vi "04 WriteOff.vi"(8 "error in (no error)":errorcluster caption="错误输入（无错误）", 11 "SerialClass 输入":refnum<class "SerialClass.lvclass">) -> (0 "error out":errorcluster caption="错误输出", 3 "SerialClass 输出":refnum<class "SerialClass.lvclass">)   [LabVIEW 2019, in "SerialClass.lvclass"]
uses:
  SerialClass.lvclass
  SerialClass.lvclass/SerialClass.ctl
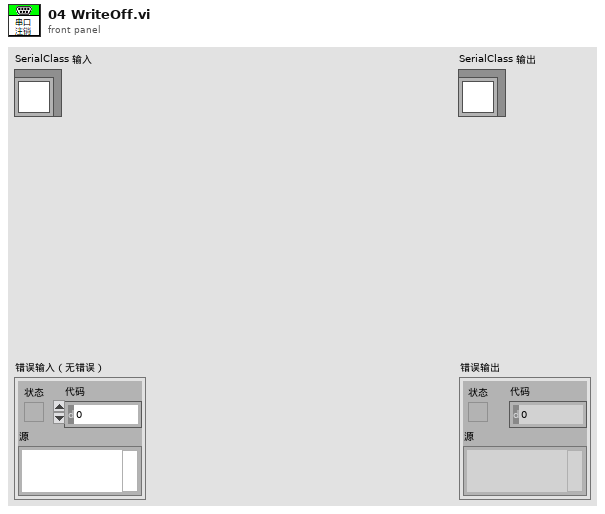
[diagram p1: front panel]
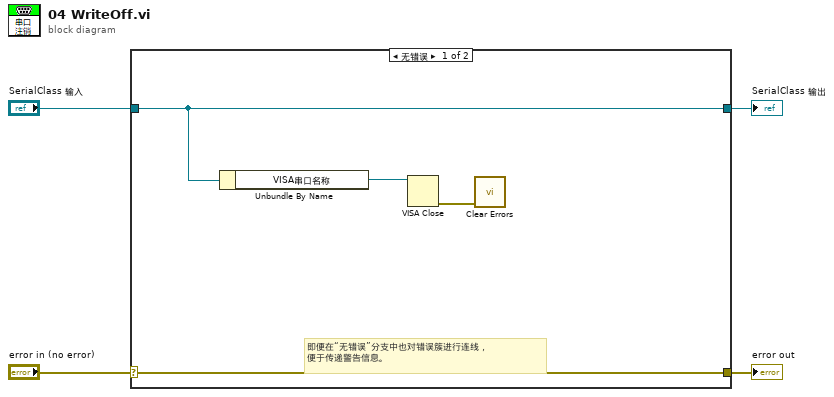
[diagram p0: block diagram]
diagram:
  n1 = case shown="无错误" "error in (no error)" {
    selector: "error in (no error)" -> [w8 w10]
    tunnel: [w8 w10] -> w3
    tunnel: [w7 w9] -> w1
    tunnel: "SerialClass 输入" -> [w7 w9]
    frame No Error {
      # "即便在“无错误”分支中也对错误簇进行连线，\n便于传递警告信息。"
      n2 = Unbundle By Name(w7) -> ("VISA串口名称"=w6:refnum<visa-resource-name>)
      n3 = VISA Close(VISA resource name=w6) -> (error out=w5:errorcluster)  [unwired: 1 in]
      n4 = call <vilib>:"Clear Errors.vi"("error in (no error)"=w5) -> ()  [unwired: 5 in, 2 out]
    }
    frame Error {
    }
  }
  "error out" <- w3
  "SerialClass 输出" <- w1
